vi "Client - Reset UI.vi"(8 "error in (no error)":errorcluster, 11 "Client - Data In":T1) -> (0 "error out":errorcluster, 3 "Client - Data Out":T1)   [LabVIEW 2024]
doc: "Resets the client user interface."
uses:
  Controls/Client/Client - Data.ctl
  Shared/Message Queue/Client Message Queues.ctl
  Shared/Message Queue/Message Cluster.ctl
  Shared/Message Queue.lvlib
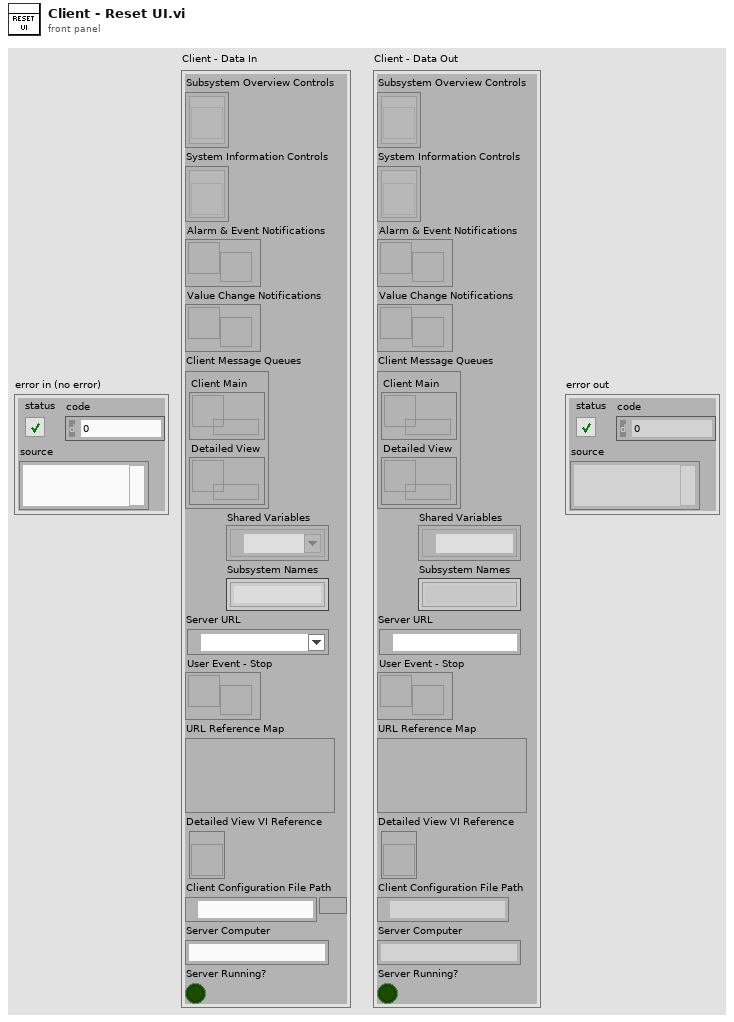
[diagram p1: front panel]
types:
  T1 = typedef "Client - Data.ctl" = cluster{"Subsystem Overview Controls":refnum<vi>[], "System Information Controls":refnum<vi>[], "Alarm & Event Notifications":refnum<user-event>, "Value Change Notifications":refnum<user-event>, "Client Message Queues":T2, "Shared Variables":refnum<k21>[], "Subsystem Names":string[], "Server URL":refnum<k21>, "User Event - Stop":refnum<user-event>, "URL Reference Map":variant, "Detailed View VI Reference":refnum<vi>, "Client Configuration File Path":path, "Server Computer":string, "Server Running?":bool}
  T2 = typedef "Message Queue.lvlib/Client Message Queues.ctl" = cluster{"Client Main":refnum<queue>, "Detailed View":refnum<queue>}
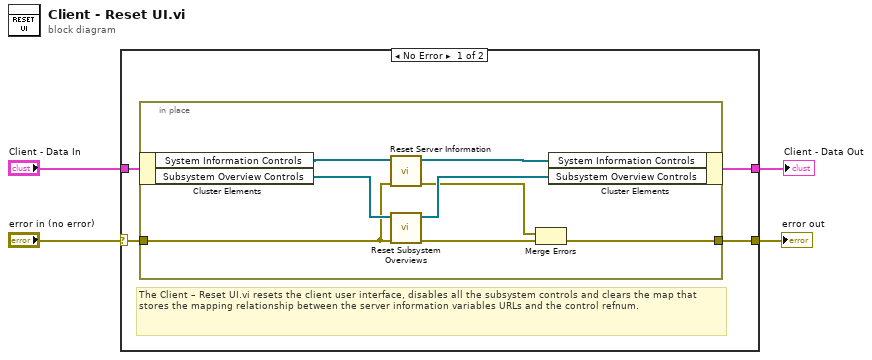
[diagram p0: block diagram]
diagram:
  n1 = case shown="No Error" "error in (no error)" {
    selector: "error in (no error)" -> [w7 w18]
    tunnel: [w5 w18] -> w3
    tunnel: "Client - Data In" -> [w8 w17]
    tunnel: [w6 w17] -> w1
    frame No Error {
      # "The Client – Reset UI.vi resets the client user interface, disables all the subsystem controls and clears the map that stores the mapping relationship between the server information variables URLs and the control refnum."
      n2 = in-place {
        in-place-border: w7 -> [w12]
        in-place-border: [w11] -> w5
        n3 = in-place-cluster #1(w8) -> ("System Information Controls"=w16:refnum<vi>[], "Subsystem Overview Controls"=w14:refnum<vi>[])
        n4 = call "Reset Server Information.vi"("error in (no error)"=w12, "System Information Controls In"=w16) -> ("error out"=w9:errorcluster, "System Information Controls Out"=w15:refnum<vi>[])  [unwired: 8 in]
        n5 = call "Reset Subsystem Overviews.vi"("error in (no error)"=w12, "Subsystem Controls In"=w14) -> ("error out"=w10:errorcluster, "Subsystem Controls Out"=w13:refnum<vi>[])  [unwired: 8 in]
        n6 = Merge Errors(w9, w10) -> (w11:errorcluster)
        n7 = in-place-cluster #1("System Information Controls"=w15, "Subsystem Overview Controls"=w13) -> (w6:T1)
      }
    }
    frame Error {
    }
  }
  "error out" <- w3
  "Client - Data Out" <- w1
